vi "ObserverDemo.vi"() -> ()   [LabVIEW 2020]
uses:
  Weather Station/Weather Station.lvclass
  ObserverFactory/ObserverFactory.lvclass
  Weather Station/Weather Station.lvclass/Weather Station.ctl
panel:
  in  "OK Button":bool
  in  "Available Notification Types":i32(listbox)
  in  "Stop Button":bool
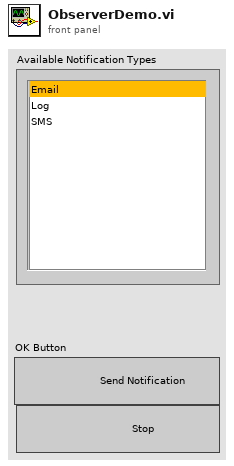
[diagram p1: front panel]
types:
  T1 = cluster{"Temperature":dbl, "Humidity":dbl, "Pressure":dbl, "Stop?":bool}
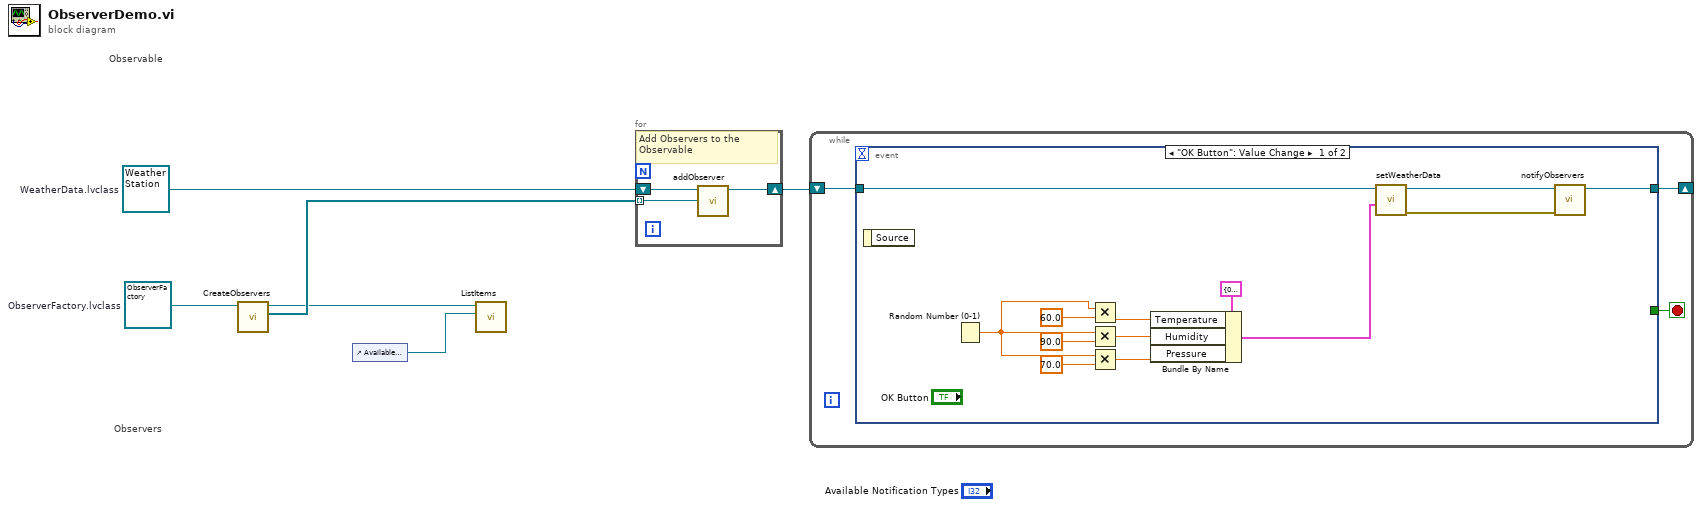
[diagram p0: block diagram]
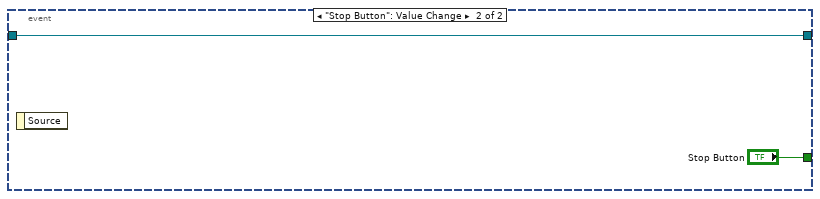
[diagram p2: hidden frame]
diagram:
  w2 = refnum<class "ObserverFactory.lvclass"> refnum  # ObserverFactory.lvclass
  w6 = refnum<class "Weather Station.lvclass"> refnum  # WeatherData.lvclass
  # "Observers"
  # "Observable"
  n1 = call "CreateObservers.vi"("ObserverFactory in"=w2) -> ("Observers"=w4:refnum<class "Observer.lvclass">[], "ObserverFactory out"=w3:refnum<class "ObserverFactory.lvclass">)  [unwired: 8 in, 1 out]
  n2 = control-ref of="Available Notification Types"() -> (w1:refnum<vi>)
  n3 = call-dynamic "ListItems.vi"("Listbox"=w1, "ObserverFactory in"=w3) -> ()  [unwired: 8 in, 2 out]
  n4 = for {
    shift-right: [w8] -> w5
    shift-left: w6 -> [w9]
    tunnel: w4 -> [w7] mode=indexing
    # "Add Observers to the Observable"
    n5 = call-dynamic "addObserver.vi"("Observer.lvclass"=w7, "Observable in"=w9) -> ("Observable out"=w8:refnum<class "Weather Station.lvclass">)  [unwired: 8 in, 1 out]
  }
  n6 = while {
    shift-right: [w11] -> _
    shift-left: w5 -> [w12]
    stop <- w10 stop-if-true
    n7 = event shown="[0] \"OK Button\": Value Change" {
      selector: _ -> [_ _]
      dyn-events: _ -> [_ _]
      timeout: _ -> [_ _]
      tunnel: w12 -> [w13 w27]
      tunnel: [w24 w27] -> w11
      tunnel: [_ "Stop Button"] -> w10
      event "OK Button": Value Change {
        n8 = event-data() -> ()  [unwired: 1 in, 1 out]
        n9 = Random Number (0-1)() -> (number: 0 to 1=w20:dbl)
        n10 = Multiply(x=w20, y=60.0) -> (x*y=w21:dbl)
        n11 = Multiply(x=w20, y=90.0) -> (x*y=w18:dbl)
        n12 = Multiply(x=w20, y=70.0) -> (x*y=w17:dbl)
        n13 = Bundle By Name(cluster=T1 {"Temperature"=0.0, "Humidity"=0.0, "Pressure"=0.0, "Stop?"=FALSE} ("WeatherData"), "Temperature"=w21, "Humidity"=w18, "Pressure"=w17) -> (w14:T1)
        n14 = call "setWeatherData.vi"("WeatherData"=w14, "WeatherData in"=w13) -> ("error out"=w22:errorcluster, "WeatherData out"=w25:refnum<class "Weather Station.lvclass">)  [unwired: 8 in]
        n15 = call-dynamic "notifyObservers.vi"("error in (no error)"=w22, "WeatherData in"=w25) -> ("WeatherData out"=w24:refnum<class "Weather Station.lvclass">)  [unwired: 8 in, 1 out]
      }
      event "Stop Button": Value Change {
        n16 = event-data() -> ()  [unwired: 1 in, 1 out]
      }
    }
  }
